vi "Th2829_Read_data.vi"(11 "VISA资源名称":refnum<visa-resource-name>) -> (2 "读取缓冲区":string, 3 "VISA资源名称 2":refnum<visa-resource-name>)   [LabVIEW 2018]
panel:
  in  "error in":errorcluster caption="错误输入（无错误）"
  out "长度":i32
  out "数值":i32
  out "返回数":u32
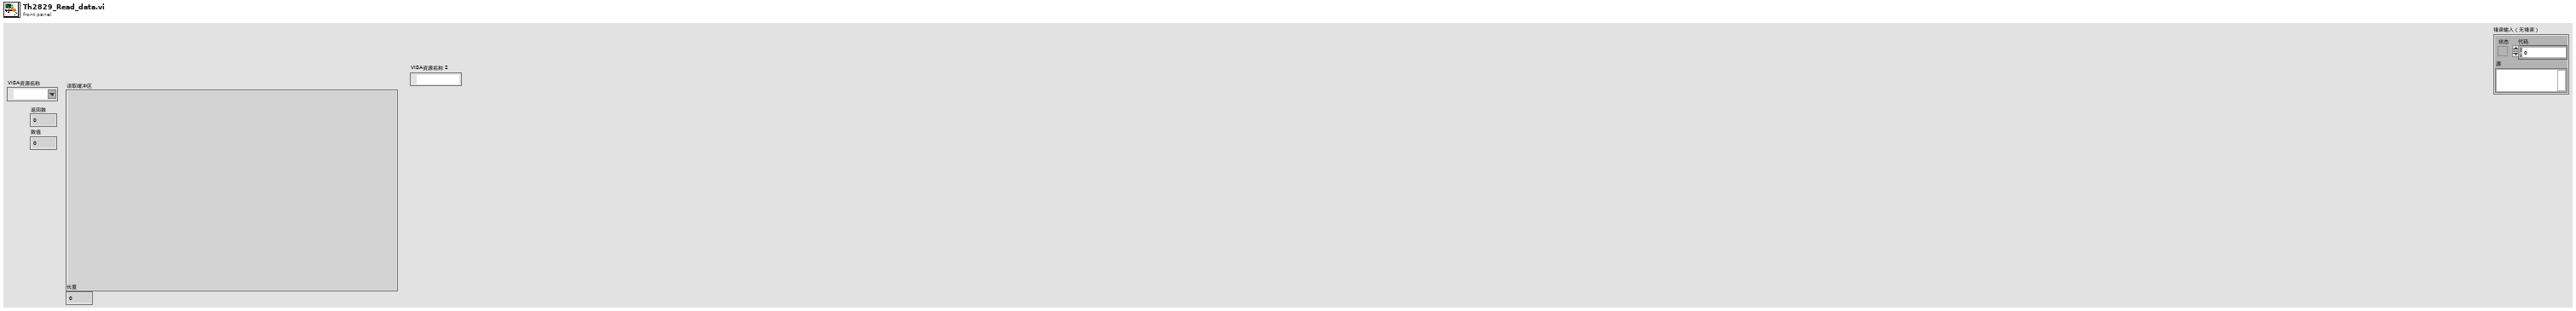
[diagram p1: front panel]
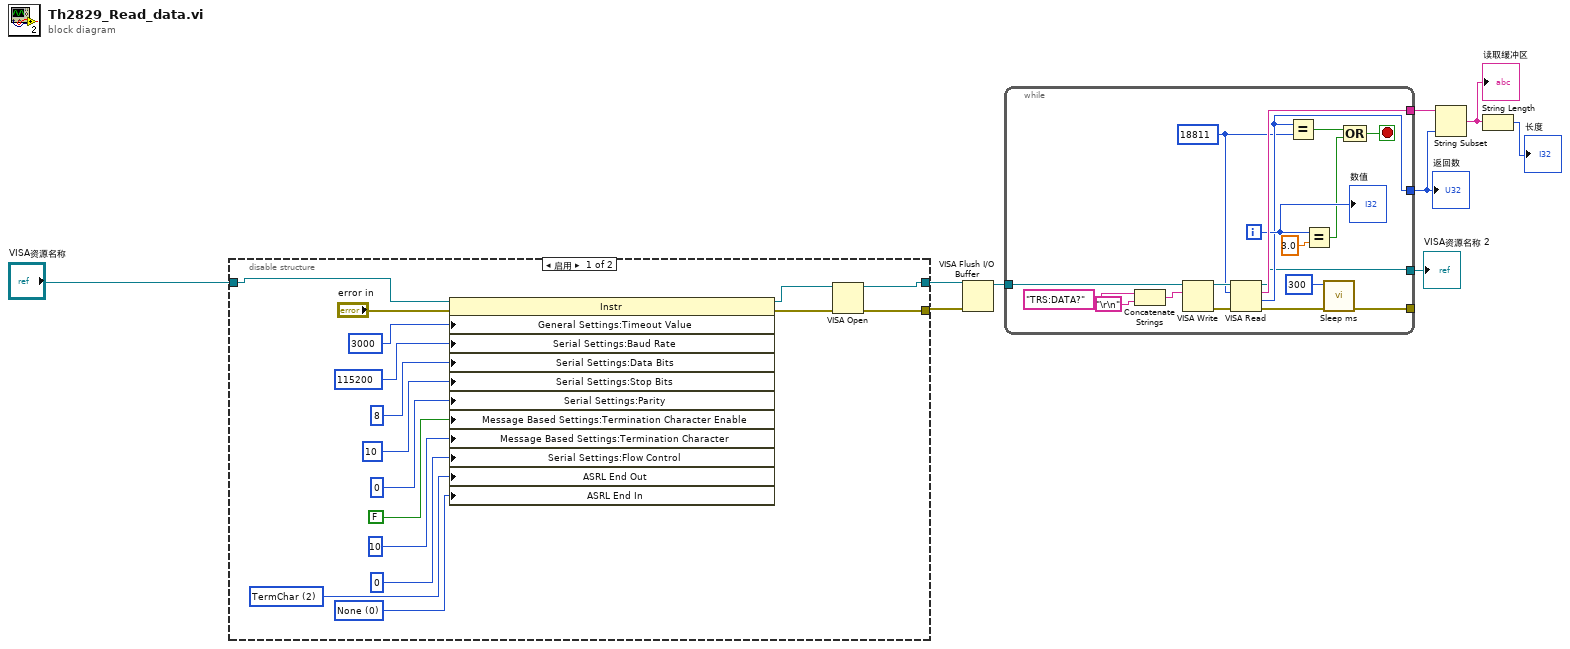
[diagram p0: block diagram]
diagram:
  n1 = disable-structure shown="启用" {
    disable-tunnel: [w25 w26] -> w3
    disable-tunnel: [w24 _] -> w2
    disable-tunnel: "VISA资源名称" -> [w21 w26]
    frame Enabled {
      w14 = u16 0 items=["None", "Last Bit", "TermChar"] ("Serial Settings:End Mode for Reads")
      w16 = u16 2 items=["None", "Last Bit", "TermChar", "Break"] ("Serial Settings:End Mode for Writes")
      n2 = property class="Instr"(reference=w21, error in="error in", "General Settings:Timeout Value"=u32 3000, "Serial Settings:Baud Rate"=u32 115200, "Serial Settings:Data Bits"=u16 8, "Serial Settings:Stop Bits"=u16 10, "Serial Settings:Parity"=u16 0, "Message Based Settings:Termination Character Enable"=FALSE ("TermChar En"), "Message Based Settings:Termination Character"=u8 10, "Serial Settings:Flow Control"=u16 0, "ASRL End Out"=w16, "ASRL End In"=w14) -> (reference out=w22:refnum<visa-resource-name>, error out=w23:errorcluster)
      n3 = VISA Open ("VISA打开")(error in (no error)=w23, VISA resource name=w22) -> (VISA resource name=w25:refnum<visa-resource-name>, error out=w24:errorcluster)  [unwired: 3 in]
    }
    frame Disabled {
    }
  }
  n4 = VISA Flush I/O Buffer(VISA resource name=w3, error in (no error)=w2) -> (VISA resource name out=w5:refnum<visa-resource-name>)  [unwired: 1 in, 1 out]
  n5 = while {
    tunnel: w5 -> [w42]
    tunnel: [w41] -> w9
    tunnel: [w35] -> w8
    tunnel: [w29] -> _
    tunnel: [w27] -> w4
    i -> [w36]
    stop <- w31 stop-if-true
    w34 = u32 18811 ("字节总数")
    n6 = Concatenate Strings("TRS:DATA?", "\r\n") -> (w38:string)
    n7 = VISA Write(VISA resource name=w42, write buffer=w38) -> (VISA resource name out=w44:refnum<visa-resource-name>, error out=w43:errorcluster)  [unwired: 1 in, 1 out]
    n8 = VISA Read(VISA resource name=w44, byte count=w34, error in (no error)=w43) -> (VISA resource name out=w27:refnum<visa-resource-name>, read buffer=w41:string, return count=w35:u32, error out=w30:errorcluster)
    n9 = Equal?(x=w35, y=w34) -> (x = y?=w33:bool)
    n10 = Equal?(x=w36, y=3.0) -> (x = y?=w32:bool)
    n11 = call "Sleep ms.vi"("error in (no error)"=w30, "等待时间（毫秒）"=u32 300) -> ("error out"=w29:errorcluster)  [unwired: 9 in]
    n12 = Compound Arithmetic op=OR ("复合运算")(w33, w32) -> (w31:bool)
    "数值" <- w36
  }
  "返回数" <- w8
  "VISA资源名称 2" <- w4
  n13 = String Subset(string=w9, length (rest)=w8) -> (substring=w7:string)  [unwired: 1 in]
  "读取缓冲区" <- w7
  n14 = String Length(string=w7) -> (length=→"长度":i32)
